vi "Data 2 Record.vi"(6 "Step":string, 9 "Time Stamp":timestamp, 10 "Data":dbl[](array[numeric])) -> (2 "Records":string)   [LabVIEW 2009]
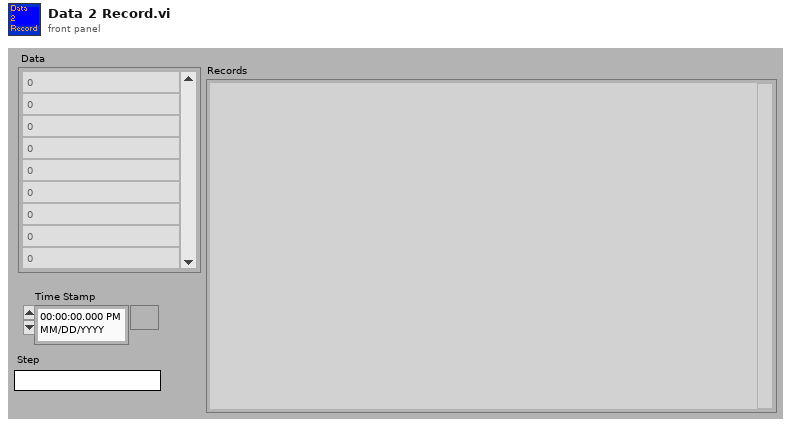
[diagram p1: front panel]
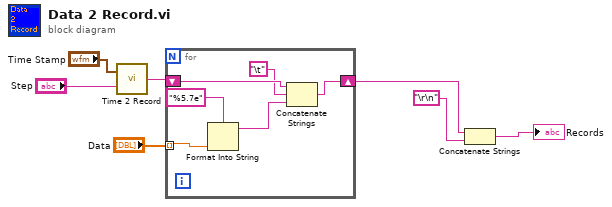
[diagram p0: block diagram]
diagram:
  n1 = call "Time 2 Record.vi"("Step"="Step", "Time Stamp"="Time Stamp") -> ("String"=w3:string)
  n2 = for {
    shift-right: [w13] -> w1
    shift-left: w3 -> [w12]
    tunnel: "Data" -> [w10] mode=indexing
    n3 = Format Into String(format string="%5.7e", w10) -> (resulting string=w9:string)  [unwired: 2 in, 1 out]
    n4 = Concatenate Strings(w12, "\t", w9) -> (w13:string)
  }
  n5 = Concatenate Strings(w1, "\r\n") -> (→"Records":string)
